vi "Check if Exist.vi"(11 "Data":variant[][](array[variant])) -> (3 "Boolean":bool)   [LabVIEW 2014]
doc: "Checks if data is valid (value not empty) which means data exists on table"
uses:
  <vilib>/addons/database/_DB Variant To Data/Database Variant To Data.xnode
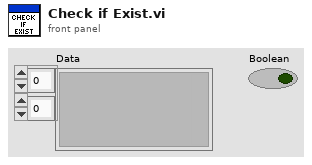
[diagram p1: front panel]
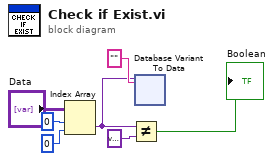
[diagram p0: block diagram]
diagram:
  n1 = Index Array(array="Data", index (row)=0, index (col)=0 ("disabled index (col)")) -> (element=w5:variant)
  n2 = Not Equal?(x=w5, y=variant) -> (x != y?=→"Boolean":bool)
  n3 = xnode "Database Variant To Data"("database variant"=w5, "type"="" ("table")) -> ()  [unwired: 1 in, 2 out]
